vi "Probe Resistance Helium (Read).vi"(6 "ISOBUS address":T3=-1 caption="ISOBUS address (-1)", 8 "error in":errorcluster, 11 "Mercury Reference In":T4) -> (0 "error out":errorcluster, 1 "Unit":T1, 2 "Resistance":dbl caption="Resistance (Ohms)", 3 "Mercury Reference Out":T4, 4 "Valid?":T2)   [LabVIEW 2013, in "Mercury iXX.lvlib" / "Level Meter.lvlib"]
doc: "Acquire the most recent resistance reading."
uses:
  <instrlib>/Mercury iXX/Public/Libraries/Level Meter.lvlib
  <instrlib>/Mercury iXX/Public/Controls/Mercury Reference.ctl
  <instrlib>/Mercury iXX/Public/Controls/Comms Transport Layer.ctl
  <instrlib>/Mercury iXX/Private/Controls/Query Dynamic Reference.ctl
  <instrlib>/Mercury iXX/Public/Controls/ISOBus Address.ctl
  <instrlib>/Mercury iXX/Public/Controls/Is Valid LED.ctl
  <instrlib>/Mercury iXX/Public/Controls/Unit String.ctl
  <instrlib>/Mercury iXX/Private/Controls/Command Verbs.ctl
  <instrlib>/Mercury iXX/Mercury iXX.lvlib
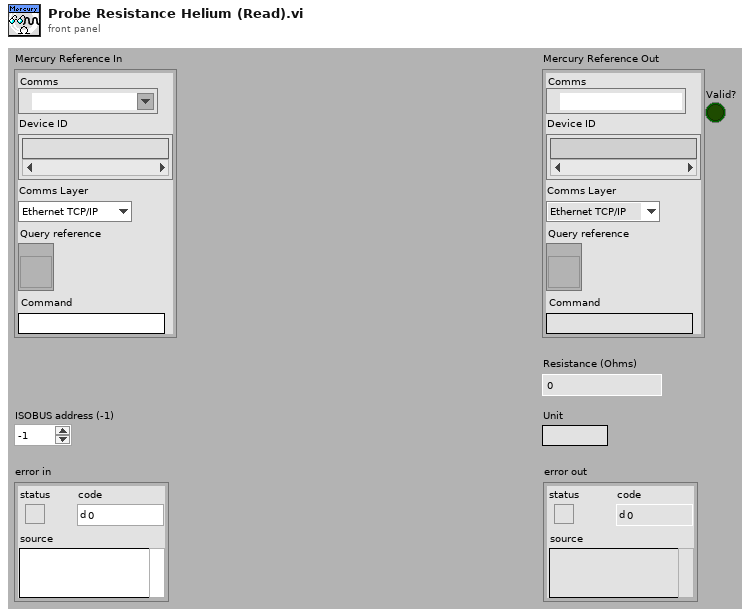
[diagram p1: front panel]
types:
  T1 = typedef "Mercury iXX.lvlib/Unit String.ctl" = string
  T2 = typedef "Mercury iXX.lvlib/Is Valid LED.ctl" = bool
  T3 = typedef "Mercury iXX.lvlib/ISOBus Address.ctl" = i32
  T4 = typedef "Mercury iXX.lvlib/Mercury Reference.ctl" = cluster{"Comms":refnum<visa-resource-name>, "Device ID":string[], "Comms Layer":T5, "Command":string, "Query reference":T6}
  T5 = typedef "Mercury iXX.lvlib/Comms Transport Layer.ctl" = enum16{"Ethernet TCP/IP", "USB", "ISOBus - RS-232", "GPIB"}
  T6 = typedef "Mercury iXX.lvlib/Query Dynamic Reference.ctl" = refnum<vi>
  T7 = typedef "Mercury iXX.lvlib/Command Verbs.ctl" = string
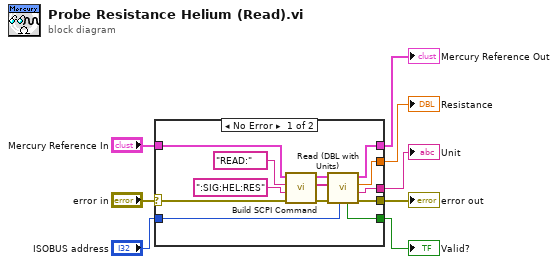
[diagram p0: block diagram]
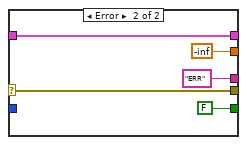
[diagram p2: hidden frame]
diagram:
  n1 = case shown="No Error" "error in" {
    selector: "error in" -> [w14 w25]
    tunnel: "Mercury Reference In" -> [w15 w26]
    tunnel: [w21 w25] -> w1
    tunnel: [w20 w26] -> w5
    tunnel: "ISOBUS address" -> [w19 _]
    tunnel: [w18 T2 FALSE ("Valid?")] -> w3
    tunnel: [w17 -inf] -> w4
    tunnel: [w16 T1 "ERR" ("Unit")] -> w2
    frame No Error {
      n2 = call <instrlib>:"Build SCPI Command.vi"("error in"=w14, "Noun(s)"=":SIG:HEL:RES" ("Command"), "Verb"=T7 "READ:", "Mercury Reference In"=w15) -> ("error out"=w10:errorcluster, "SCPI Message(s)"=w9:string[], "Mercury Reference Out"=w13:T4)  [unwired: 5 out]
      n3 = call <instrlib>:"Read (DBL with Units).vi"("ISOBUS address"=w19, "error in"=w10, "SCPI Message(s)"=w9, "Mercury Reference In"=w13) -> ("error out"=w21:errorcluster, "Unit"=w16:T1, "Data (Dbl)"=w17:dbl, "Mercury Reference Out"=w20:T4, "Valid?"=w18:T2)  [unwired: 3 out]
    }
    frame Error {
    }
  }
  "Mercury Reference Out" <- w5
  "error out" <- w1
  "Valid?" <- w3
  "Unit" <- w2
  "Resistance" <- w4
